vi "Get Image.vi"(1 "Input Picture":picture, 2 "String":string="mario_standing.png", 3 "Bottom":i32, 4 "Left":i32) -> (0 "Main Picture":picture)   [LabVIEW 2014]
panel:
  out "right":i32
  out "left":i32
  out "bottom":i32
  out "top":i32
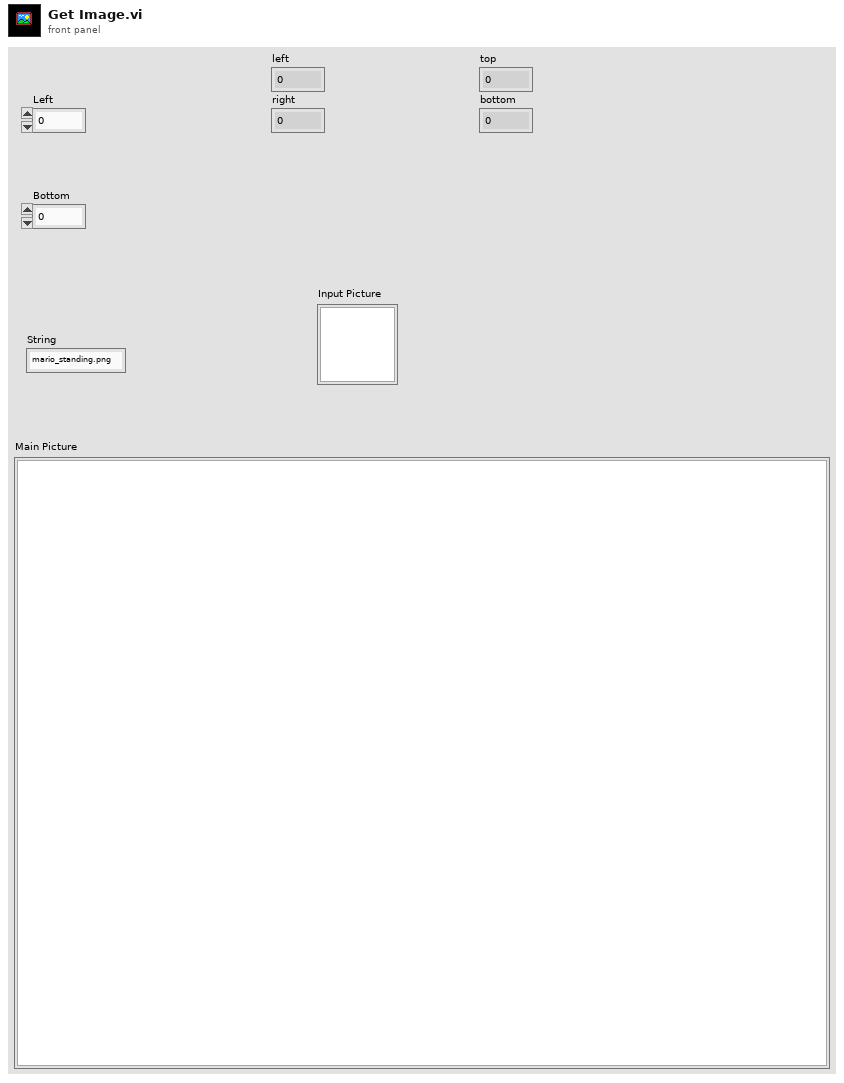
[diagram p1: front panel]
types:
  T1 = typedef "imagedata.ctl" = cluster{"image type":i32, "image depth":i32, "image":u8[], "mask":u8[], "colors":u32[], "Rectangle":cluster{"left":i16, "top":i16, "right":i16, "bottom":i16}}
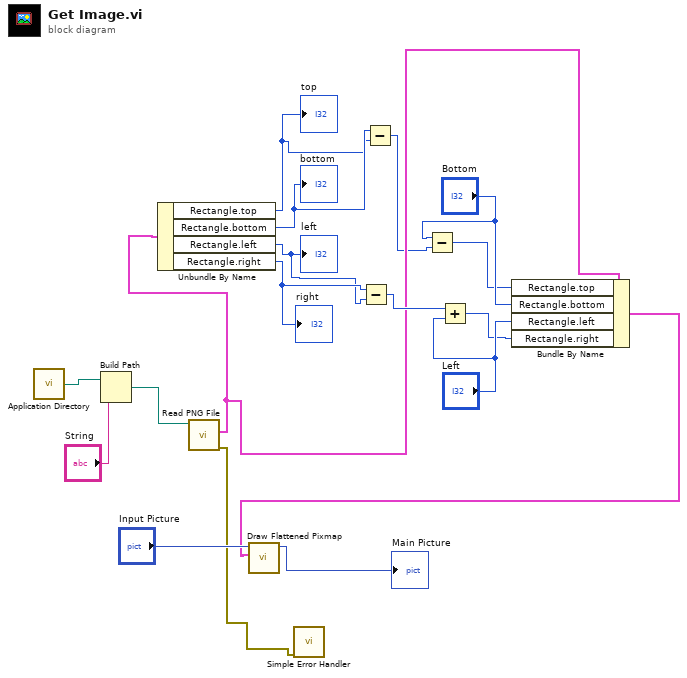
[diagram p0: block diagram]
diagram:
  n1 = call <vilib>:"Application Directory.vi"() -> ("Application Directory"=w15:path)
  n2 = Build Path(base path=w15, name or relative path="String") -> (appended path=w17:path)
  n3 = call <vilib>:"Read PNG File.vi"("path to PNG file"=w17) -> ("error out"=w13:errorcluster, "image data"=w5:T1)  [unwired: 8 in, 1 out]
  n4 = Unbundle By Name(w5) -> ("Rectangle.top"=w11:i16, "Rectangle.bottom"=w12:i16, "Rectangle.left"=w9:i16, "Rectangle.right"=w10:i16)
  "top" <- w11
  "bottom" <- w12
  "left" <- w9
  "right" <- w10
  n5 = call <vilib>:"Simple Error Handler.vi"("error in (no error)"=w13) -> ()  [unwired: 4 in, 5 out]
  n6 = Subtract(x=w10, y=w9) -> (x-y=w8:i16)
  n7 = Subtract(x=w12, y=w11) -> (x-y=w2:i16)
  n8 = Subtract(x="Bottom", y=w2) -> (x-y=w1:i32)
  n9 = Add(x=w8, y="Left") -> (x+y=w6:i32)
  n10 = Bundle By Name(cluster=w5, "Rectangle.top"=w1, "Rectangle.bottom"="Bottom", "Rectangle.left"="Left", "Rectangle.right"=w6) -> (w4:T1)
  n11 = call <vilib>:"Draw Flattened Pixmap.vi"("image data"=w4, "picture"="Input Picture") -> ("new picture"=→"Main Picture":picture)  [unwired: 7 in]
